vi "Initialize.vi"(8 "error in (no error)":errorcluster, 11 "AnalogDiscoveryFunction in":refnum<class "AnalogDiscoveryFunction.lvclass">) -> (0 "error out":errorcluster, 3 "AnalogDiscoveryFunction out":refnum<class "AnalogDiscoveryFunction.lvclass">)   [LabVIEW 2020, in "AnalogDiscoveryFunction.lvclass"]
doc: "VIRTUAL FUNCTION\n\nThis VI should be overwritten by methods using the specific initialization procedure for the respective child class."
uses:
  AnalogDiscoveryFunction.lvclass
  AnalogDiscoveryFunction.lvclass/AnalogDiscoveryFunction.ctl
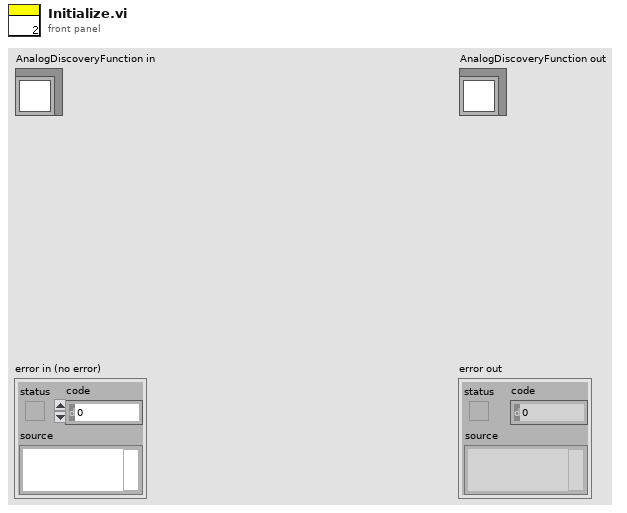
[diagram p1: front panel]
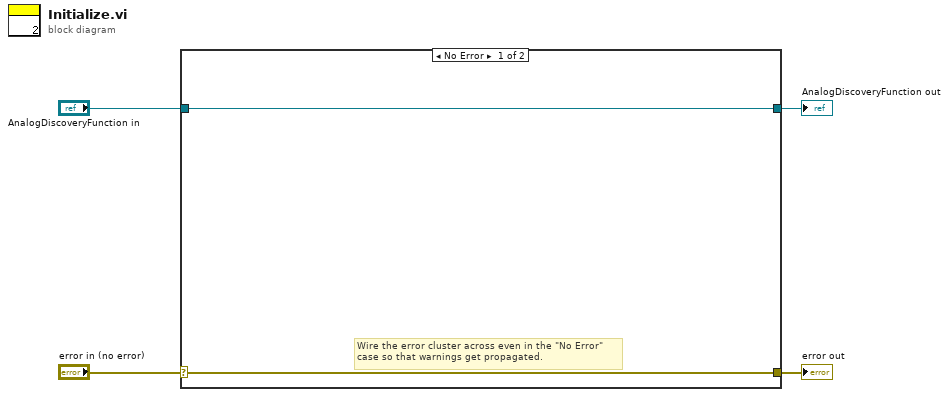
[diagram p0: block diagram]
diagram:
  n1 = case shown="No Error" "error in (no error)" {
    selector: "error in (no error)" -> [w5 w8]
    tunnel: [w5 w8] -> w3
    tunnel: [w6 w7] -> w1
    tunnel: "AnalogDiscoveryFunction in" -> [w6 w7]
    frame No Error {
      # "Wire the error cluster across even in the \"No Error\"\ncase so that warnings get propagated."
    }
    frame Error {
    }
  }
  "error out" <- w3
  "AnalogDiscoveryFunction out" <- w1
